vi "Autonomous State global.vi"() -> ()   [LabVIEW 2014]
uses:
  Autonomous Play State.ctl
  Autonomous Commands/Autonomous Command Names.ctl
panel:
  out "Autonomous Execution State":T1
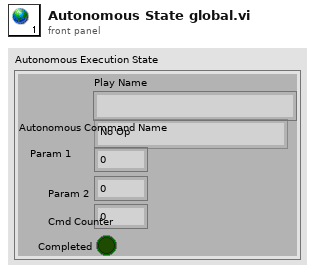
[diagram p1: front panel]
types:
  T1 = typedef "Autonomous Play State.ctl" = cluster{"Play Name":string, "Autonomous Command Name":T2, "Param 1":dbl, "Param 2":dbl, "Cmd Counter":i32, "Completed":bool}
  T2 = typedef "Autonomous Command Names.ctl" = enum16{"No Op", "Drive Distance Robot", "Drive Time Robot", "Translate Distance Robot", "Translate Time Robot", "Drive Distance Field", "Drive Time Field", "Translate Distance Field", "Translate Time Field", "Rotate Robot", "Set Initial Gyro Value", "Lifter to Setpoint", "Wait", "Do Not use", "Drive Distance Field (Gyro Hold)", "Translate Distance Field (Gyro Hold)", "Can", "Grabber", "Drive Distance Field (Sensor Stop, Gyro Hold)", "Move Direction Field (Gyro Hold)", "Rotate Robot 90 about Tote", "Reset Gyro", "Find Tote", "Get Tote Into Robot", "Lower Can Grabber"}
diagram:
